vi "Configure Channel Output.vi"(8 "error in (no error)":errorcluster, 9 "Output (0: Channel Display)":u16(ring) items=["Channel Display", "X or Y"], 10 "Channel (1: Channel 1)":u16(ring)=1 items=["Channel 1"=1, "Channel 2"=2], 11 "VISA resource name":refnum<visa-resource-name>) -> (0 "error out":errorcluster, 3 "VISA resource name out":refnum<visa-resource-name>)   [LabVIEW 2015, in "Stanford Research 830.lvlib"]
doc: "Configures the channel output of the instrument."
uses:
  <instrlib>/Stanford Research 830/Stanford Research 830.lvlib
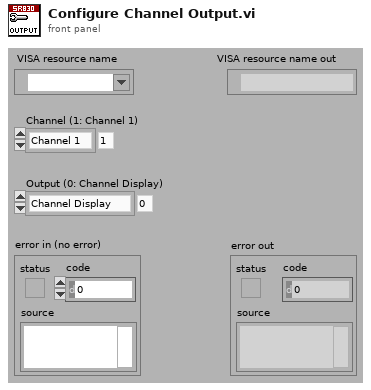
[diagram p1: front panel]
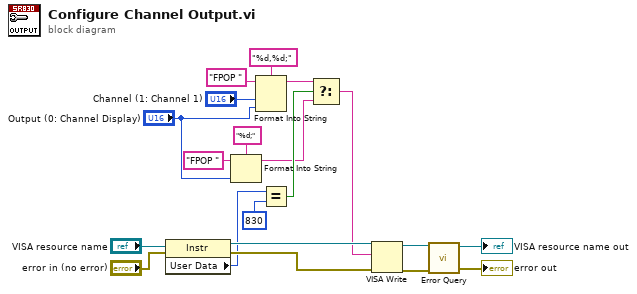
[diagram p0: block diagram]
diagram:
  n1 = property class="Instr"(reference="VISA resource name", error in="error in (no error)") -> (reference out=w11:refnum<visa-resource-name>, error out=w10:errorcluster, "User Data"=w9:u32)
  n2 = Format Into String(format string="%d;", initial string="FPOP ", "Output (0: Channel Display)") -> (resulting string=w2:string)  [unwired: 1 in, 1 out]
  n3 = Format Into String(format string="%d,%d;", initial string="FPOP ", "Channel (1: Channel 1)", "Output (0: Channel Display)") -> (resulting string=w6:string)  [unwired: 1 in, 1 out]
  n4 = Equal?(x=w9, y=u32 830) -> (x = y?=w7:bool)
  n5 = Select(t=w6, s=w7, f=w2) -> (s? t:f=w1:string)
  n6 = VISA Write(VISA resource name=w11, write buffer=w1, error in (no error)=w10) -> (VISA resource name out=w15:refnum<visa-resource-name>, error out=w14:errorcluster)  [unwired: 1 out]
  n7 = call <instrlib>:"Error Query.vi"("error in (no error)"=w14, "VISA resource name"=w15) -> ("error out"=→"error out":errorcluster, "VISA resource name out"=→"VISA resource name out":refnum<visa-resource-name>)  [unwired: 7 in, 1 out]
